vi "QBridge_65.vi"() -> (0 "error":errorcluster)   [LabVIEW 2012]
uses:
  <vilib>/Instr/_visa.llb/VISA Configure Serial Port (Instr).vi
panel:
  out "Status":string
  out "Command":string
  in  "base port number":u16=54200
  in  "address":string="200.131.64.236"
  out "listener ID":refnum<k5>
  out "serial ref":refnum<visa-resource-name>
  out "RS232":bool
  in  "stop bits":u16(ring)=10 items=["1.0"=10, "1.5"=15, "2.0"=20]
  in  "flow control":u16(ring) items=["None", "XON/XOFF", "RTS/CTS", "XON/XOFF & RTS/CTS", "DTR/DSR", "XON/XOFF & DTR/DSR"]
  in  "parity":enum16{"None", "Odd", "Even", "Mark", "Space"}(ring)
  in  "baud rate":u32=2400
  in  "VISA resource name":refnum<visa-resource-name>="COM65"
  in  "data bits":u16=8 min=5 max=8 step=1
  out "TCP/IP":bool
  out "connection ID":refnum<k5>
  in  "stop":bool
  # "QBRIDGE"
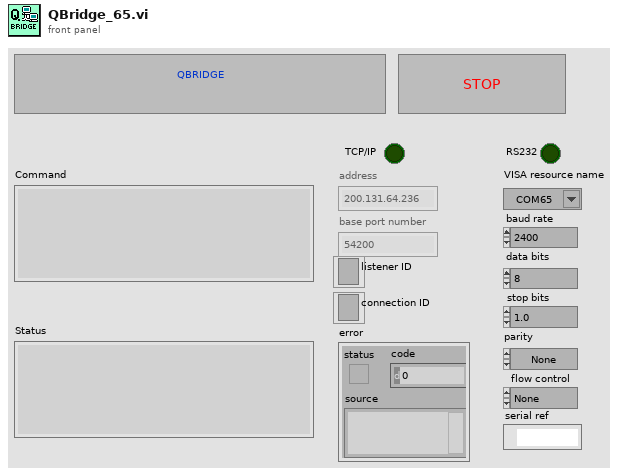
[diagram p1: front panel]
types:
  T1 = enum16{"Standard", "Buffered", "CRLF", "Immediate"}
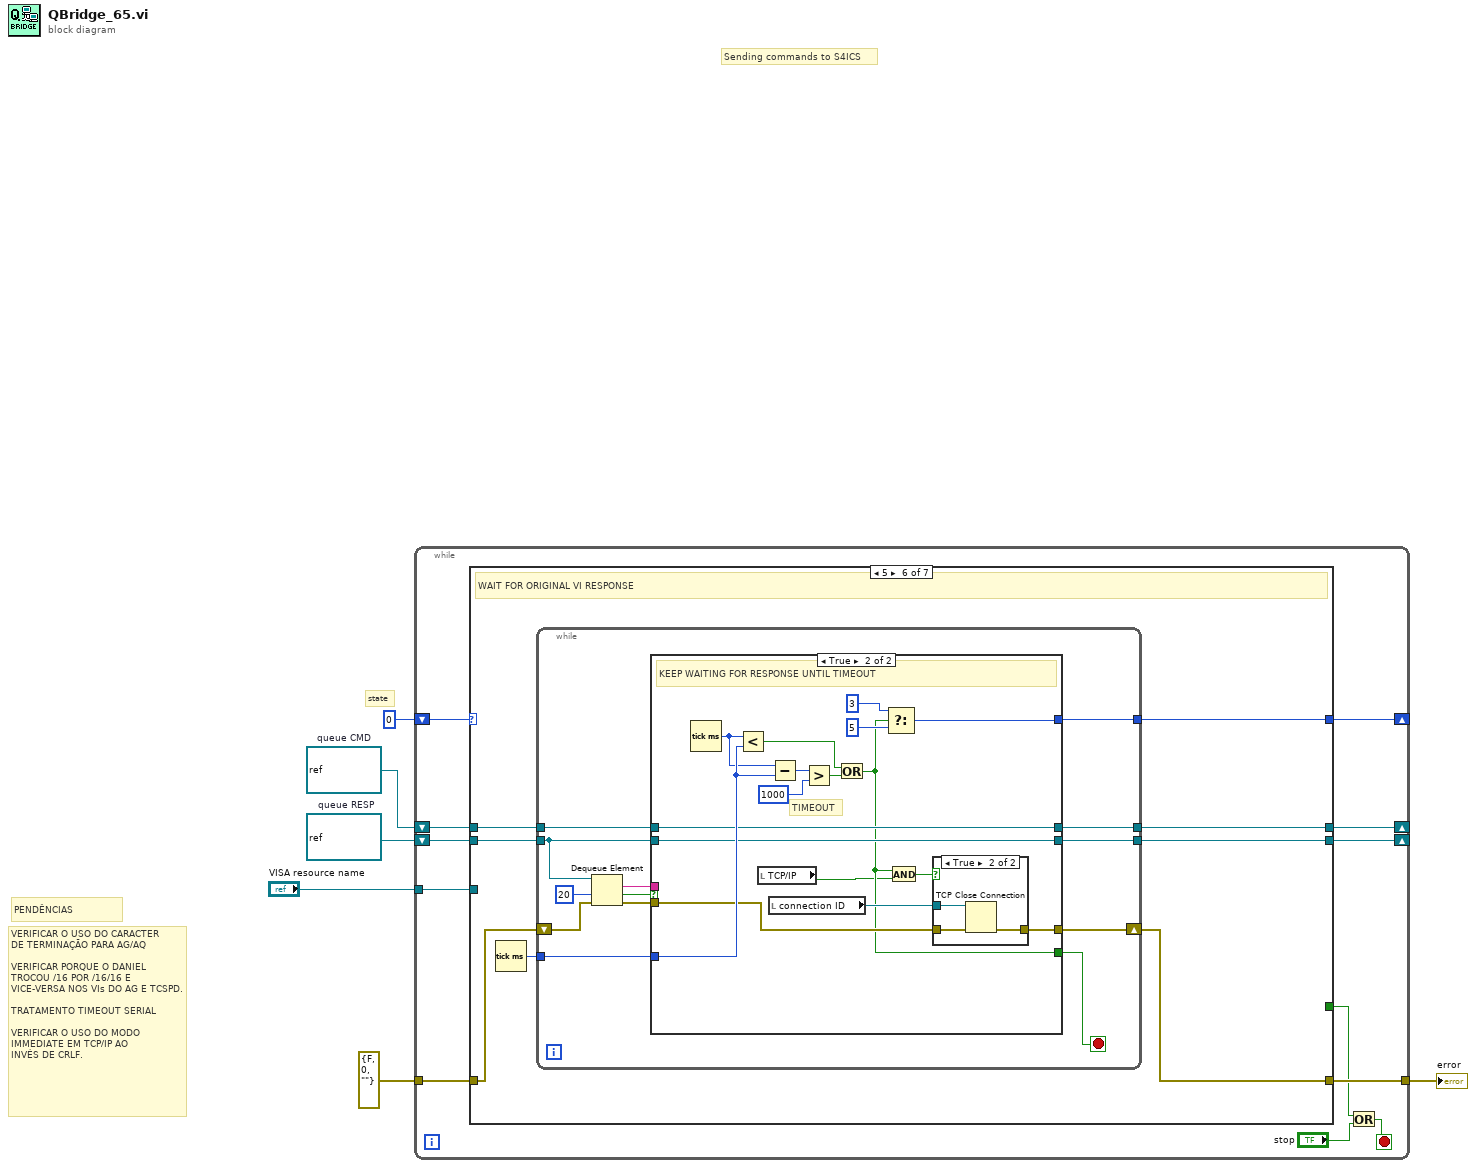
[diagram p0: block diagram]
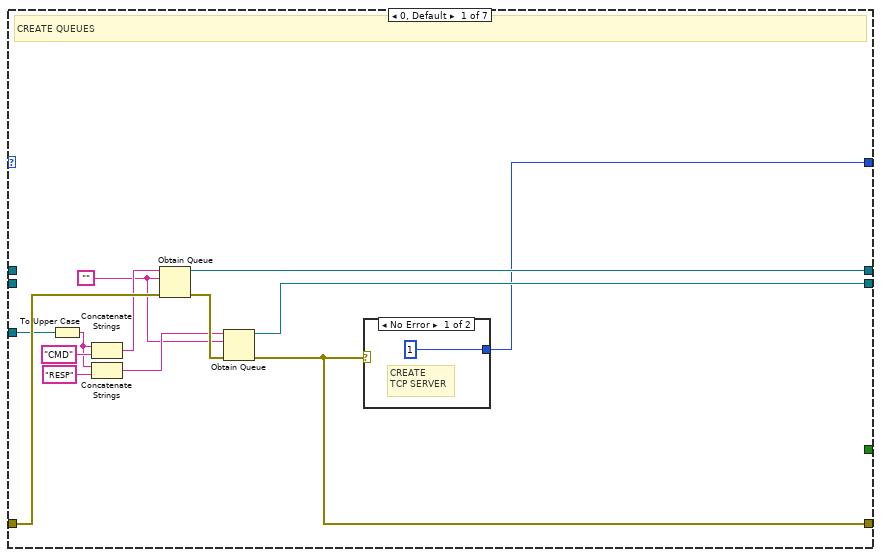
[diagram p2: hidden frame]
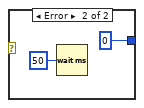
[diagram p3: hidden frame]
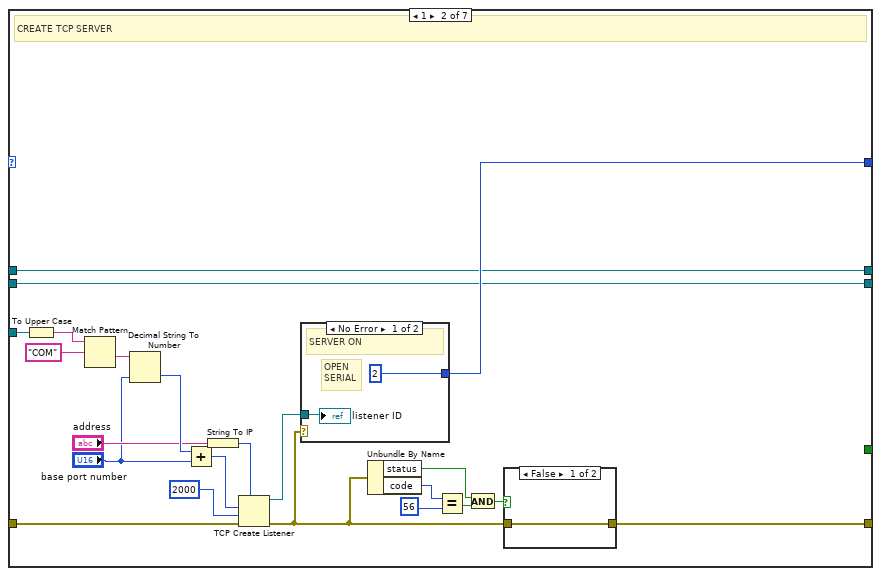
[diagram p4: hidden frame]
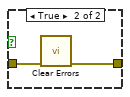
[diagram p5: hidden frame]
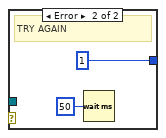
[diagram p6: hidden frame]
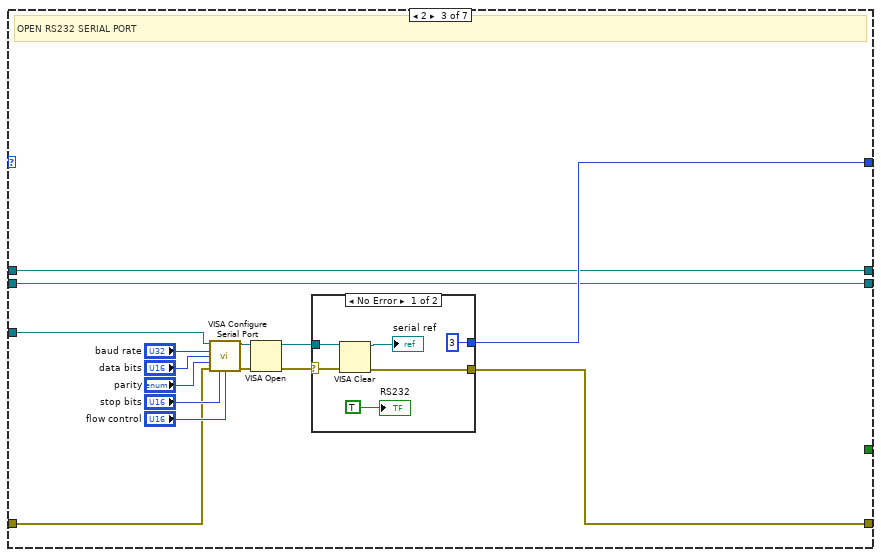
[diagram p7: hidden frame]
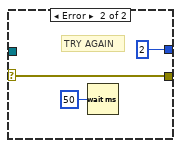
[diagram p8: hidden frame]
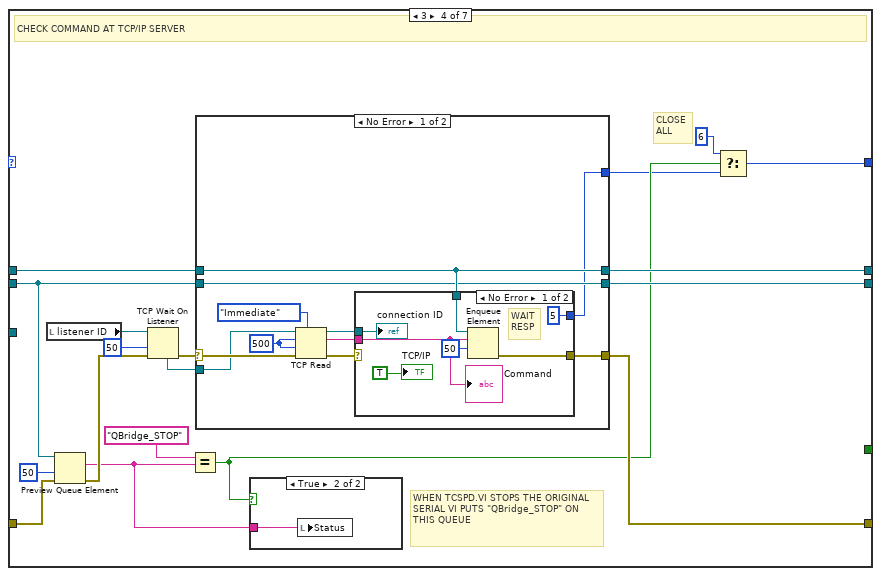
[diagram p9: hidden frame]
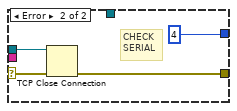
[diagram p11: hidden frame]
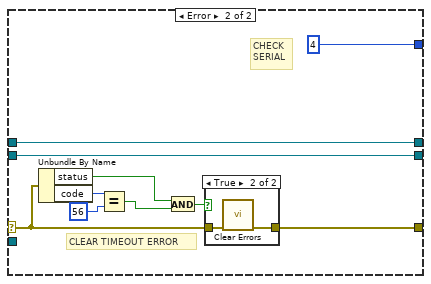
[diagram p12: hidden frame]
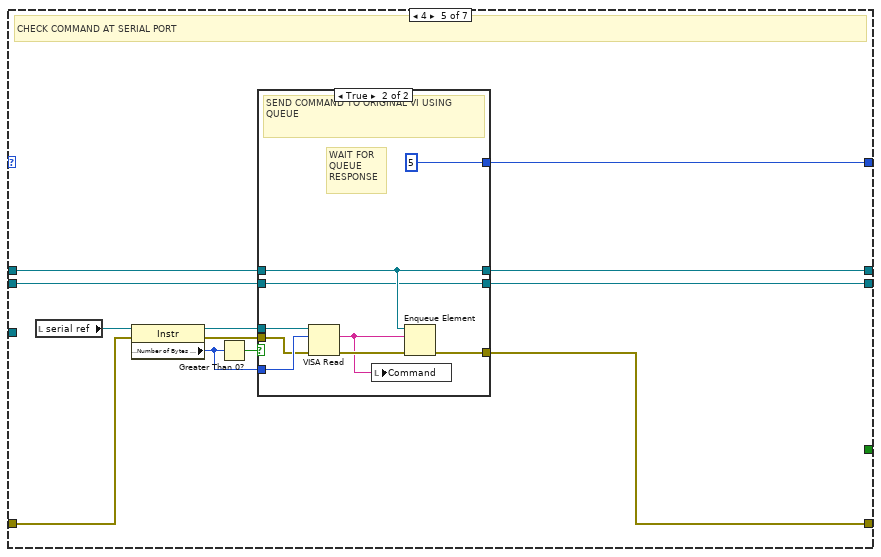
[diagram p14: hidden frame]
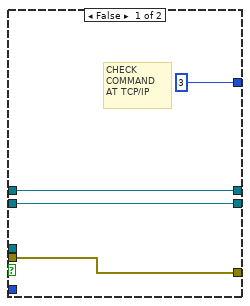
[diagram p15: hidden frame]
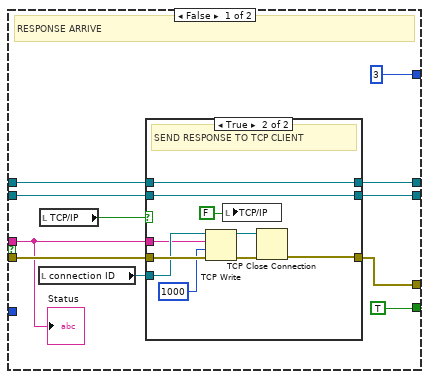
[diagram p16: hidden frame]
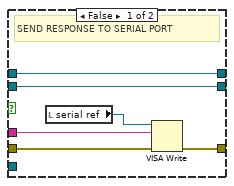
[diagram p17: hidden frame]
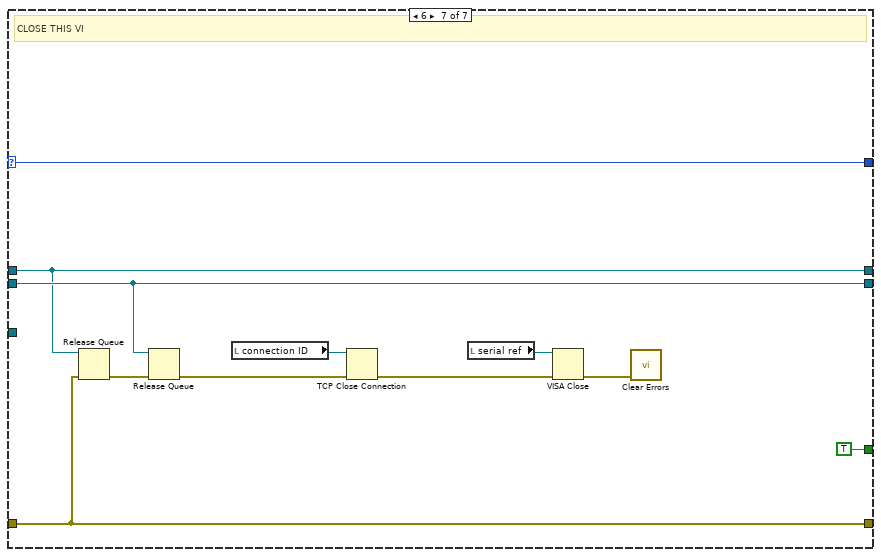
[diagram p19: hidden frame]
diagram:
  w2 = refnum<queue> refnum  # queue RESP
  w1 = refnum<queue> refnum  # queue CMD
  # "PENDÊNCIAS"
  # "VERIFICAR O USO DO CARACTER\nDE TERMINAÇÃO PARA AG/AQ\n\nVERIFICAR PORQUE O DANIEL  TROCOU /16 POR /16/16 E VICE-VERSA NOS VIs DO AG E TCSPD.\n\nTRATAMENTO TIMEOUT SERIAL\n\nVERIFICAR O USO DO MODO \nIMMEDIATE EM TCP/IP AO\nINVÉS DE CRLF."
  # "state"
  # "Sending commands to S4ICS"
  n1 = while {
    shift-right: [w16] -> _
    shift-left: u16 0 -> [w18]
    tunnel: "VISA resource name" -> [w11]
    shift-right: [w10] -> _
    shift-left: w1 -> [w8]
    shift-right: [w9] -> _
    shift-left: w2 -> [w7]
    tunnel: errorcluster {"status"=FALSE, "code"=0, "source"=""} ("error in (no error)") -> [w17]
    tunnel: [w15] -> w4
    stop <- w13 stop-if-true
    n2 = case shown="5" w18 {
      selector: w18 -> [_ _ _ _ _ _ w246]
      tunnel: w17 -> [w28 w54 w72 w105 w152 w173 w240]
      tunnel: [w29 w53 w66 w94 w143 w171 w246] -> w16
      tunnel: [w26 w52 w68 w98 w142 w167 w240] -> w15
      tunnel: [w31 w43 w65 w99 w144 w168 w243] -> w10
      tunnel: [w30 w44 w64 w100 w145 w169 w244] -> w9
      tunnel: [_ _ _ _ _ _ TRUE] -> w12
      tunnel: w11 -> [w25 w50 w67 _ _ _ _]
      tunnel: w8 -> [_ w43 w65 w101 w147 w170 w243]
      tunnel: w7 -> [_ w44 w64 w96 w146 w174 w244]
      frame 0, Default {
        w19 = ""
        # "CREATE QUEUES"
        n3 = To Upper Case(1:w25) -> (0:w20:string)
        n4 = Concatenate Strings(w20, "CMD" ("string")) -> (w21:string)
        n5 = Concatenate Strings(w20, "RESP" ("string")) -> (w23:string)
        n6 = Obtain Queue(name (unnamed)=w21, element data type=w19, error in (no error)=w28) -> (queue out=w31:refnum<queue>, error out=w27:errorcluster)  [unwired: 2 in, 1 out]
        n7 = Obtain Queue(name (unnamed)=w23, element data type=w19, error in (no error)=w27) -> (queue out=w30:refnum<queue>, error out=w26:errorcluster)  [unwired: 2 in, 1 out]
        n8 = case shown="No Error" w26 {
          tunnel: [u16 1 u16 0] -> w29
          frame No Error {
            # "CREATE\nTCP SERVER"
          }
          frame Error {
            n9 = Wait (ms)(milliseconds to wait=u32 50) -> ()  [unwired: 1 out]
          }
        }
      }
      frame 1 {
        # "CREATE TCP SERVER"
        n10 = To Upper Case(1:w50) -> (0:w48:string)
        n11 = Match Pattern(string=w48, regular expression="COM") -> (after substring=w47:string)  [unwired: 1 in, 3 out]
        n12 = Decimal String To Number(string=w47, default (0L)="base port number") -> (number=w46:u16)  [unwired: 1 in, 1 out]
        n13 = Add(x=w46, y="base port number") -> (x+y=w45:u16)
        n14 = String To IP(1:"address") -> (0:w51:u32)
        n15 = TCP Create Listener(7:w51, 8:w54, 9:2000 ("timeout ms (60000)"), 10:w45) -> (0:w40:errorcluster, 3:w56:refnum<k5>)  [unwired: 1 in, 1 out]
        n16 = case shown="No Error" w40 {
          tunnel: [u16 2 u16 1] -> w53
          tunnel: w56 -> [w60 _]
          frame No Error {
            # "OPEN\nSERIAL"
            # "SERVER ON"
            "listener ID" <- w60
          }
          frame Error {
            # "TRY AGAIN"
            n17 = Wait (ms)(milliseconds to wait=u32 50) -> ()  [unwired: 1 out]
          }
        }
        n18 = Unbundle By Name(w40) -> ("status"=w35:bool, "code"=w39:i32)
        n19 = Equal?(x=w39, y=56 ("code")) -> (x = y?=w36:bool)
        n20 = And(x=w35, y=w36) -> (x .and. y?=w37:bool)
        n21 = case shown="False" w37 {
          tunnel: w40 -> [w57 w59]
          tunnel: [w57 w58] -> w52
          frame False {
          }
          frame True {
            n22 = call <vilib>:"Clear Errors.vi"("error in (no error)"=w59) -> ("error out"=w58:errorcluster)  [unwired: 6 in]
          }
        }
      }
      frame 2 {
        # "OPEN RS232 SERIAL PORT"
        n23 = call-poly "VISA Configure Serial Port"("VISA resource name"=w67, "baud rate (9600)"="baud rate", "data bits (8)"="data bits", "parity (0:none)"="parity", "error in (no error)"=w72, "stop bits (10: 1 bit)"="stop bits", "flow control (0:none)"="flow control") -> ("VISA resource name out"=w70:refnum<visa-resource-name>, "error out"=w71:errorcluster)  [unwired: 7 in]
        n24 = VISA Open(error in (no error)=w71, VISA resource name=w70) -> (VISA resource name=w78:refnum<visa-resource-name>, error out=w69:errorcluster)  [unwired: 3 in]
        n25 = case shown="No Error" w69 {
          selector: w69 -> [w83 w87]
          tunnel: w78 -> [w84 _]
          tunnel: [w82 w87] -> w68
          tunnel: [u16 3 u16 2] -> w66
          frame No Error {
            n26 = VISA Clear(VISA resource name=w84, error in (no error)=w83) -> (VISA resource name out=→"serial ref":refnum<visa-resource-name>, error out=w82:errorcluster)
            "RS232" <- TRUE ("RS232")
          }
          frame Error {
            # "TRY AGAIN"
            n27 = Wait (ms)(milliseconds to wait=u32 50) -> ()  [unwired: 1 out]
          }
        }
      }
      frame 3 {
        # "WHEN TCSPD.VI STOPS THE ORIGINAL SERIAL VI PUTS \"QBridge_STOP\" ON THIS QUEUE"
        # "CLOSE\nALL"
        # "CHECK COMMAND AT TCP/IP SERVER"
        n28 = local read "listener ID"() -> (w104:refnum<k5>)
        n29 = Preview Queue Element(queue=w96, timeout in ms (-1)=50, error in (no error)=w105) -> (element=w92:string, error out=w97:errorcluster)  [unwired: 2 out]
        n30 = TCP Wait On Listener(8:w97, 9:50 ("timeout ms (wait forever: -1)"), 11:w104) -> (0:w102:errorcluster, 4:w95:refnum<k5>)  [unwired: 1 in, 3 out]
        n31 = Equal?(x="QBridge_STOP", y=w92) -> (x = y?=w93:bool)
        n32 = case shown="No Error" w102 {
          selector: w102 -> [w117 w134]
          tunnel: [w113 w138] -> w98
          tunnel: [w107 u16 4] -> w89
          tunnel: w101 -> [w114 w136]
          tunnel: w96 -> [w111 w135]
          tunnel: [w111 w135] -> w100
          tunnel: [w114 w136] -> w99
          tunnel: w95 -> [w109 _]
          frame No Error {
            w115 = 500 ("timeout ms (25000)")
            n33 = TCP Read(connection ID=w109, bytes to read=w115, error in (no error)=w117, 7:T1."Immediate" ("mode (standard)"), 9:w115) -> (connection ID out=w112:refnum<k5>, data out=w110:string, error out=w108:errorcluster)
            n34 = case shown="No Error" w108 {
              selector: w108 -> [_ w127]
              tunnel: w114 -> [w124 _]
              tunnel: [w123 w125] -> w113
              tunnel: w112 -> [w122 w126]
              tunnel: w110 -> [w119 _]
              tunnel: [u16 5 u16 4] -> w107
              frame No Error {
                # "WAIT\nRESP"
                n35 = Enqueue Element(queue=w124, element=w119, timeout in ms (-1)=50) -> (error out=w123:errorcluster)  [unwired: 1 in, 2 out]
                "connection ID" <- w122
                "TCP/IP" <- TRUE
                "Command" <- w119
              }
              frame Error {
                # "CHECK\nSERIAL"
                n36 = TCP Close Connection(connection ID=w126, error in (no error)=w127) -> (error out=w125:errorcluster)  [unwired: 1 in, 1 out]
              }
            }
          }
          frame Error {
            # "CHECK\nSERIAL"
            # "CLEAR TIMEOUT ERROR"
            n37 = Unbundle By Name(w134) -> ("status"=w129:bool, "code"=w133:i32)
            n38 = Equal?(x=w133, y=56 ("specific error code to clear (0: all)")) -> (x = y?=w130:bool)
            n39 = And(x=w129, y=w130) -> (x .and. y?=w131:bool)
            n40 = case shown="True" w131 {
              tunnel: w134 -> [w139 w141]
              tunnel: [w139 w140] -> w138
              frame False {
              }
              frame True {
                n41 = call <vilib>:"Clear Errors.vi"("error in (no error)"=w141) -> ("error out"=w140:errorcluster)  [unwired: 6 in]
              }
            }
          }
        }
        n42 = case shown="True" w93 {
          tunnel: w92 -> [_ w106]
          frame False {
          }
          frame True {
            n43 = local write "Status"(w106) -> ()
          }
        }
        n44 = Select(t=u16 6, s=w93, f=w89) -> (s? t:f=w94:u16)
      }
      frame 4 {
        # "CHECK COMMAND AT SERIAL PORT"
        n45 = local read "serial ref"() -> (w153:refnum<visa-resource-name>)
        n46 = property class="Instr"(reference=w153, error in=w152) -> (reference out=w150:refnum<visa-resource-name>, error out=w149:errorcluster, "Serial Settings:Number of Bytes at Serial Port"=w148:u32)
        n47 = Greater Than 0?(x=w148) -> (x > 0?=w151:bool)
        n48 = case shown="True" w151 {
          tunnel: w150 -> [_ w166]
          tunnel: w149 -> [w154 w161]
          tunnel: w148 -> [_ w165]
          tunnel: w147 -> [w156 w164]
          tunnel: w146 -> [w157 w160]
          tunnel: [w157 w160] -> w145
          tunnel: [w156 w164] -> w144
          tunnel: [u16 3 u16 5] -> w143
          tunnel: [w154 w162] -> w142
          frame False {
            # "CHECK\nCOMMAND\nAT TCP/IP"
          }
          frame True {
            # "WAIT FOR\nQUEUE\nRESPONSE"
            # "SEND COMMAND TO ORIGINAL VI USING QUEUE"
            n49 = VISA Read(VISA resource name=w166, byte count=w165, error in (no error)=w161) -> (read buffer=w158:string, error out=w159:errorcluster)  [unwired: 2 out]
            n50 = local write "Command"(w158) -> ()
            n51 = Enqueue Element(queue=w164, element=w158, error in (no error)=w159) -> (error out=w162:errorcluster)  [unwired: 1 in, 2 out]
          }
        }
      }
      frame 5 {
        # "WAIT FOR ORIGINAL VI RESPONSE"
        n52 = Tick Count (ms)() -> (millisecond timer value=w172:u32)
        n53 = while {
          tunnel: w174 -> [w179]
          tunnel: w172 -> [w182]
          tunnel: [w180] -> w171
          tunnel: w170 -> [w178]
          tunnel: [w177] -> w169
          tunnel: [w176] -> w168
          shift-right: [w175] -> w167
          shift-left: w173 -> [w183]
          stop <- w181 stop-if-true
          n54 = Dequeue Element(queue=w179, timeout in ms (-1)=20, error in (no error)=w183) -> (element=w186:string, timed out?=w185:bool, error out=w184:errorcluster)  [unwired: 1 out]
          n55 = case shown="True" w185 {
            tunnel: w184 -> [w192 w220]
            tunnel: w186 -> [w188 _]
            tunnel: [u16 3 w225] -> w180
            tunnel: w182 -> [_ w231]
            tunnel: [TRUE w217] -> w181
            tunnel: w179 -> [w195 w222]
            tunnel: w178 -> [w196 w221]
            tunnel: [w193 w222] -> w177
            tunnel: [w194 w221] -> w176
            tunnel: [w190 w219] -> w175
            frame False {
              # "RESPONSE ARRIVE"
              n56 = local read "connection ID"() -> (w191:refnum<k5>)
              n57 = local read "TCP/IP"() -> (w197:bool)
              n58 = case shown="True" w197 {
                tunnel: w196 -> [w199 w214]
                tunnel: w195 -> [w200 w213]
                tunnel: [w199 w214] -> w194
                tunnel: [w200 w213] -> w193
                tunnel: w188 -> [w202 w210]
                tunnel: w192 -> [w203 w212]
                tunnel: w191 -> [_ w211]
                tunnel: [w201 w206] -> w190
                frame False {
                  # "SEND RESPONSE TO SERIAL PORT"
                  n59 = local read "serial ref"() -> (w204:refnum<visa-resource-name>)
                  n60 = VISA Write(VISA resource name=w204, write buffer=w202, error in (no error)=w203) -> (error out=w201:errorcluster)  [unwired: 2 out]
                }
                frame True {
                  # "SEND RESPONSE TO TCP CLIENT"
                  n61 = TCP Write(connection ID=w211, data in=w210, error in (no error)=w212, 9:1000 ("timeout ms (25000)")) -> (connection ID out=w207:refnum<k5>, error out=w208:errorcluster)  [unwired: 1 out]
                  n62 = local write "TCP/IP"(FALSE) -> ()
                  n63 = TCP Close Connection(connection ID=w207, error in (no error)=w208) -> (error out=w206:errorcluster)  [unwired: 1 in, 1 out]
                }
              }
              "Status" <- w188
            }
            frame True {
              # "TIMEOUT"
              # "KEEP WAITING FOR RESPONSE UNTIL TIMEOUT"
              n64 = Tick Count (ms)() -> (millisecond timer value=w230:u32)
              n65 = Less?(x=w230, y=w231) -> (x < y?=w226:bool)
              n66 = local read "TCP/IP"() -> (w216:bool)
              n67 = local read "connection ID"() -> (w218:refnum<k5>)
              n68 = Subtract(x=w230, y=w231) -> (x-y=w229:u32)
              n69 = Greater?(x=w229, y=u32 1000 ("millisecond timer value")) -> (0:w227:bool)
              n70 = Or(x=w226, y=w227) -> (x .or. y?=w217:bool)
              n71 = Select(t=u16 3, s=w217, f=u16 5) -> (s? t:f=w225:u16)
              n72 = And(x=w217, y=w216) -> (x .and. y?=w215:bool)
              n73 = case shown="True" w215 {
                tunnel: w220 -> [w232 w235]
                tunnel: [w232 w234] -> w219
                tunnel: w218 -> [_ w233]
                frame False {
                }
                frame True {
                  n74 = TCP Close Connection(connection ID=w233, error in (no error)=w235) -> (error out=w234:errorcluster)  [unwired: 1 in, 1 out]
                }
              }
            }
          }
        }
      }
      frame 6 {
        # "CLOSE THIS VI"
        n75 = Release Queue(queue=w243, error in (no error)=w240) -> (error out=w239:errorcluster)  [unwired: 1 in, 2 out]
        n76 = Release Queue(queue=w244, error in (no error)=w239) -> (error out=w238:errorcluster)  [unwired: 1 in, 2 out]
        n77 = local read "connection ID"() -> (w242:refnum<k5>)
        n78 = TCP Close Connection(connection ID=w242, error in (no error)=w238) -> (error out=w237:errorcluster)  [unwired: 1 in, 1 out]
        n79 = local read "serial ref"() -> (w241:refnum<visa-resource-name>)
        n80 = VISA Close(VISA resource name=w241, error in (no error)=w237) -> (error out=w236:errorcluster)
        n81 = call <vilib>:"Clear Errors.vi"("error in (no error)"=w236) -> ()  [unwired: 6 in, 1 out]
      }
    }
    n82 = Or(x=w12, y="stop") -> (x .or. y?=w13:bool)
  }
  "error" <- w4
